vi "Create EventReport.vi"(6 "Verbose":bool, 8 "error in (no error)":errorcluster, 10 "Report Event":refnum<user-event>, 11 "Test Report.Event in":refnum<class "Test Report.Event.lvclass">) -> (0 "error out":errorcluster, 3 "Test Report.Event out":refnum<class "Test Report.Event.lvclass">)   [LabVIEW 2013, in "Caraya.lvlib" / "Test Report.Event.lvclass"]
uses:
  Test Report.Event.lvclass
  Test Report/Test Report.lvclass/Test Report.ctl
  Test Report/Test Report.lvclass
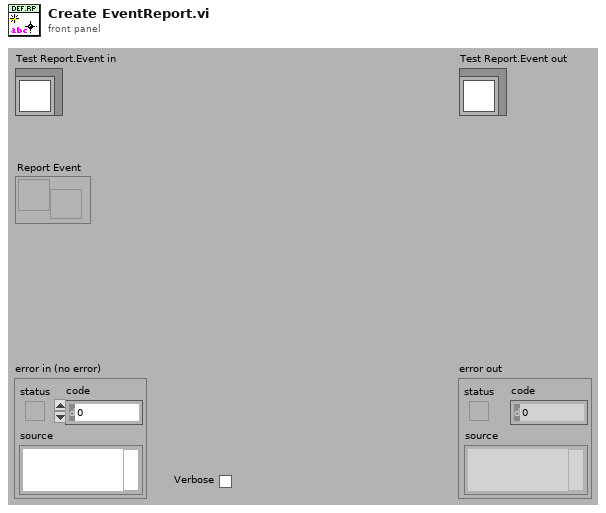
[diagram p1: front panel]
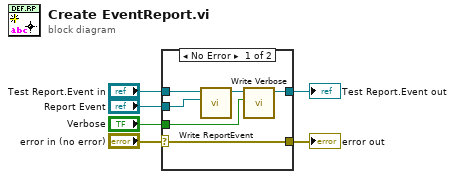
[diagram p0: block diagram]
diagram:
  n1 = case shown="No Error" "error in (no error)" {
    selector: "error in (no error)" -> [w10 w13]
    tunnel: "Test Report.Event in" -> [w12 w14]
    tunnel: [w8 w14] -> w5
    tunnel: "Report Event" -> [w11 _]
    tunnel: [w10 w13] -> w2
    tunnel: "Verbose" -> [w7 _]
    frame No Error {
      n2 = call "Write ReportEvent.vi"("Report Event"=w11, "Test Report.Default in"=w12) -> ("Test Report.Default out"=w9:refnum<class "Test Report.Event.lvclass">)  [unwired: 9 in]
      n3 = call "Write Verbose.vi"("Verbose"=w7, "Test Report in"=w9) -> ("Test Report out"=w8:refnum<class "Test Report.Event.lvclass">)  [unwired: 8 in, 1 out]
    }
    frame Error {
    }
  }
  "error out" <- w2
  "Test Report.Event out" <- w5
